vi "LHe Convert %-liters (No Objects).vi"(10 "L":dbl, 11 "%":dbl) -> (2 "%out":dbl, 3 "Lout":dbl)   [LabVIEW 2009]
panel:
  in  "arraylevels":cluster{"%":dbl, "L":dbl}[](array[cluster])=[{"%"=0.0, "L"=0.5}, {"%"=5.0, "L"=1.0}, {"%"=10.0, "L"=1.6}, {"%"=15.0, "L"=2.2}, {"%"=20.0, "L"=2.7}, {"%"=25.0, "L"=3.3}, {"%"=30.0, "L"=3.9}, {"%"=35.0, "L"=4.8}, {"%"=40.0, "L"=6.2}, {"%"=45.0, "L"=7.7}, {"%"=50.0, "L"=9.1}, {"%"=55.0, "L"=10.6}, {"%"=60.0, "L"=12.0}, {"%"=65.0, "L"=13.4}, {"%"=70.0, "L"=14.9}, {"%"=75.0, "L"=16.4}, {"%"=80.0, "L"=17.8}, {"%"=85.0, "L"=19.2}, {"%"=90.0, "L"=20.7}, {"%"=95.0, "L"=22.2}, {"%"=100.0, "L"=23.2}]
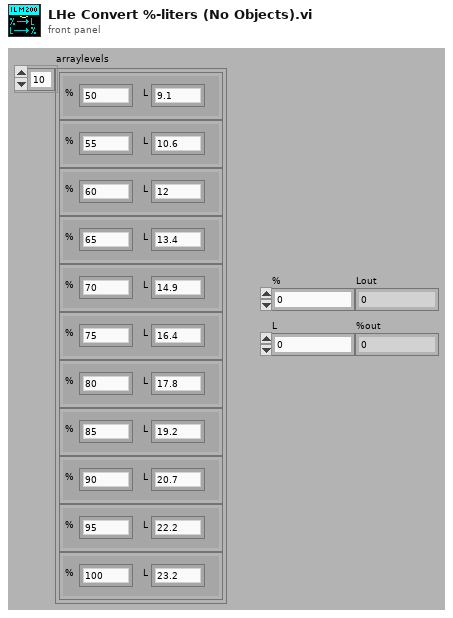
[diagram p1: front panel]
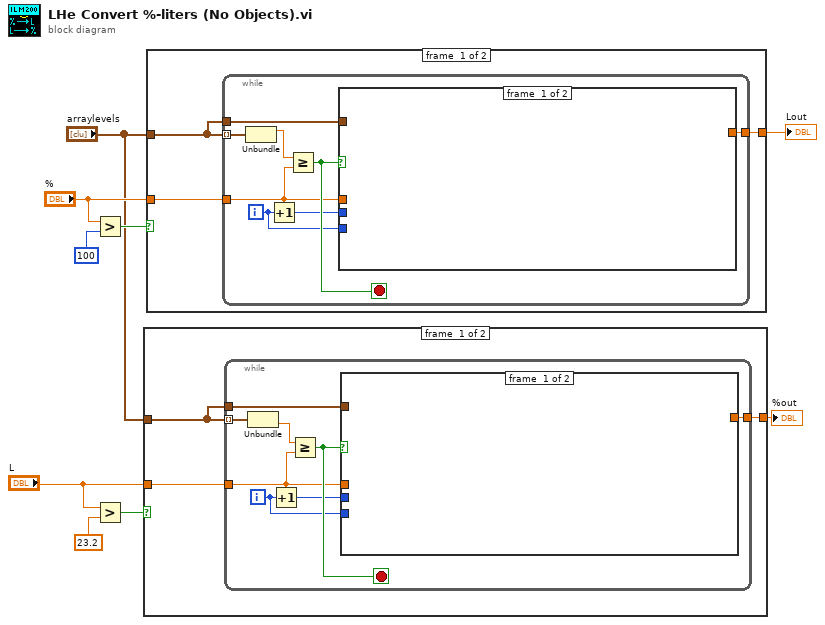
[diagram p0: block diagram]
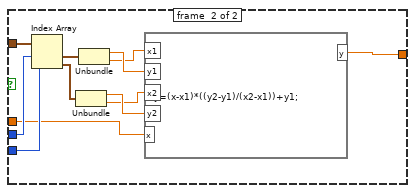
[diagram p2: hidden frame]
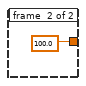
[diagram p3: hidden frame]
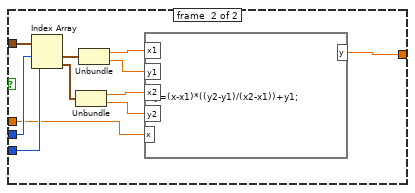
[diagram p4: hidden frame]
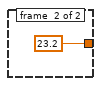
[diagram p5: hidden frame]
diagram:
  n1 = Greater?(x="%", y=100) -> (0:w7:bool)
  n2 = Greater?(x="L", y=23.2) -> (0:w3:bool)
  n3 = case shown="True" w3 {
    tunnel: "L" -> [w12 _]
    tunnel: "arraylevels" -> [w11 _]
    tunnel: [w10 100.0] -> w1
    frame #0 {
      n4 = while {
        tunnel: w11 -> [w20] mode=indexing
        tunnel: w12 -> [w15]
        tunnel: w11 -> [w18]
        tunnel: [w13] -> w10
        i -> [w16]
        stop <- w19 stop-if-true
        n5 = Unbundle(w20) -> ("L"=w14:dbl)  [unwired: 1 out]
        n6 = Increment(x=w16) -> (x+1=w17:i32)
        n7 = Greater Or Equal?(x=w14, y=w15) -> (x >= y?=w19:bool)
        n8 = case shown="False" w19 {
          tunnel: w18 -> [_ w31]
          tunnel: w17 -> [_ w30]
          tunnel: w16 -> [_ w28]
          tunnel: w15 -> [_ w26]
          tunnel: [_ w21] -> w13
          frame #0 {
          }
          frame #1 {
            n9 = Index Array(array=w31, index #1=w30, index #2=w28) -> (element #1=w29:cluster{"%":dbl, "L":dbl}, element #2=w27:cluster{"%":dbl, "L":dbl})
            n10 = Unbundle(w27) -> ("%"=w23:dbl, "L"=w22:dbl)
            n11 = Unbundle(w29) -> ("%"=w25:dbl, "L"=w24:dbl)
            n12 = formula code="y=(x-x1)*((y2-y1)/(x2-x1))+y1;"("x1"=w24, "x2"=w22, "y1"=w25, "y2"=w23, "x"=w26) -> ("y"=w21:dbl)
          }
        }
      }
    }
    frame #1 {
    }
  }
  "%out" <- w1
  n13 = case shown="True" w7 {
    tunnel: "%" -> [w35 _]
    tunnel: "arraylevels" -> [w34 _]
    tunnel: [w33 23.2] -> w2
    frame #0 {
      n14 = while {
        tunnel: w34 -> [w43] mode=indexing
        tunnel: w35 -> [w37]
        tunnel: w34 -> [w40]
        tunnel: [w36] -> w33
        i -> [w38]
        stop <- w41 stop-if-true
        n15 = Unbundle(w43) -> ("%"=w42:dbl)  [unwired: 1 out]
        n16 = Increment(x=w38) -> (x+1=w39:i32)
        n17 = Greater Or Equal?(x=w42, y=w37) -> (x >= y?=w41:bool)
        n18 = case shown="False" w41 {
          tunnel: w40 -> [_ w54]
          tunnel: w39 -> [_ w53]
          tunnel: w38 -> [_ w49]
          tunnel: w37 -> [_ w45]
          tunnel: [_ w44] -> w36
          frame #0 {
          }
          frame #1 {
            n19 = Index Array(array=w54, index #1=w53, index #2=w49) -> (element #1=w52:cluster{"%":dbl, "L":dbl}, element #2=w48:cluster{"%":dbl, "L":dbl})
            n20 = Unbundle(w48) -> ("%"=w47:dbl, "L"=w46:dbl)
            n21 = Unbundle(w52) -> ("%"=w51:dbl, "L"=w50:dbl)
            n22 = formula code="y=(x-x1)*((y2-y1)/(x2-x1))+y1;"("x1"=w51, "x2"=w47, "y1"=w50, "y2"=w46, "x"=w45) -> ("y"=w44:dbl)
          }
        }
      }
    }
    frame #1 {
    }
  }
  "Lout" <- w2
